vi "Write OpCfg to GXML File.vi"(8 "error in (no error)":errorcluster, 10 "Write?":bool, 11 "XML File Path":path) -> (0 "error out":errorcluster, 3 "XML String Out":string)   [LabVIEW 2015, in "Tool Cfg.lvlib"]
uses:
  Tool Cfg.lvlib
  _Tool OpCfg GXML Format Cluster--typedef.ctl
  ConfigGLOB.vi
  <vilib>/NI/GXML/GXML.lvlib
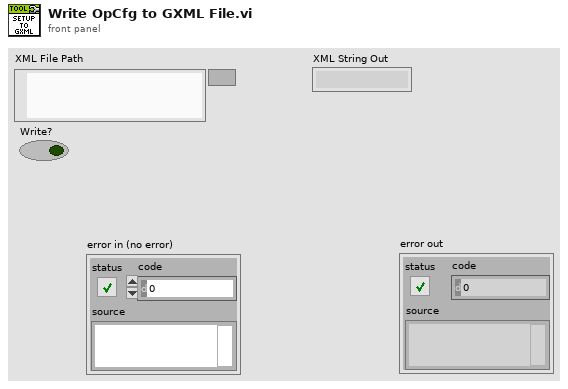
[diagram p1: front panel]
types:
  T1 = typedef "Tool Cfg.lvlib/_Tool OpCfg GXML Format Cluster--typedef.ctl" = cluster{"Use Tool Cfg":bool, "Use Tool Cal":bool, "Fake Data":bool, "Mode":i16, "Array Subset Length":i16, "nArrays to Read":i16, "Full Array Read Length":i16, "nSubarraysPerSensor":i16}
  T2 = typedef "Tool Cfg.lvlib/_Tool Operation Config Cluster--typedef.ctl" = cluster{"Use Tool Cfg":bool, "Use Tool Cal":bool, "Fake Data?":bool, "Mode":i16, "Array Subset Length":i16, "nArrays to Read":i16, "Full Array Read Length":i16, "nSubarrays/Sensor":i16}
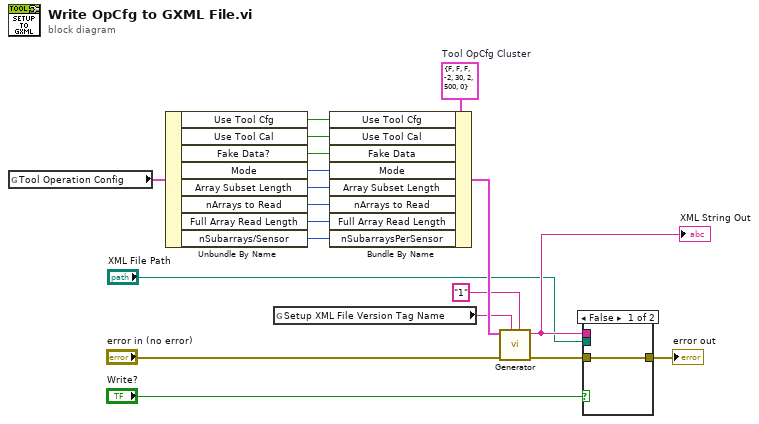
[diagram p0: block diagram]
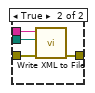
[diagram p2: hidden frame]
diagram:
  w18 = T1 {"Use Tool Cfg"=FALSE, "Use Tool Cal"=FALSE, "Fake Data"=FALSE, "Mode"=-2, "Array Subset Length"=30, "nArrays to Read"=2, "Full Array Read Length"=500, "nSubarraysPerSensor"=0}  # Tool OpCfg Cluster
  n1 = global read "ConfigGLOB.vi" "Tool Operation Config"() -> (w19:T2)
  n2 = Unbundle By Name(w19) -> ("Use Tool Cfg"=w17:bool, "Use Tool Cal"=w16:bool, "Fake Data?"=w15:bool, "Mode"=w14:i16, "Array Subset Length"=w13:i16, "nArrays to Read"=w12:i16, "Full Array Read Length"=w11:i16, "nSubarrays/Sensor"=w10:i16)
  n3 = global read "ConfigGLOB.vi" "Setup XML File Version Tag Name"() -> (w5:string)
  n4 = Bundle By Name(cluster=w18, "Use Tool Cfg"=w17, "Use Tool Cal"=w16, "Fake Data"=w15, "Mode"=w14, "Array Subset Length"=w13, "nArrays to Read"=w12, "Full Array Read Length"=w11, "nSubarraysPerSensor"=w10) -> (w9:T1)
  n5 = call <vilib>:"Generator.vi"("Version String"="1", "Version Tag Name"=w5, "error in"="error in (no error)", "Variant"=w9) -> ("error out"=w7:errorcluster, "XML String Out"=w3:string)  [unwired: 6 in]
  "XML String Out" <- w3
  n6 = case shown="False" "Write?" {
    tunnel: w7 -> [w20 w24]
    tunnel: [w20 w23] -> w6
    tunnel: w3 -> [_ w22]
    tunnel: "XML File Path" -> [_ w21]
    frame False {
    }
    frame True {
      n7 = call <vilib>:"Write XML to File.vi"("error in"=w24, "XML File Path"=w21, "XML Input"=w22) -> ("error out"=w23:errorcluster)  [unwired: 8 in]
    }
  }
  "error out" <- w6
